vi "Init Loop Data.vi"(7 "VolatusAPI":refnum<class "VolatusAPI.lvclass">, 8 "error in (no error)":refnum<class "MultiErrors.lvclass">, 9 "Sequencer":refnum<class "MessageQ.lvclass">, 10 "Sequence Config":refnum<class "Sequence Config.lvclass">, 11 "Sequence in":refnum<class "Sequence.lvclass">) -> (0 "error out":refnum<class "MultiErrors.lvclass">, 2 "Loop Data":T1, 3 "Sequence out":refnum<class "Sequence.lvclass">, 5 "Period":i64)   [LabVIEW 2023, in "VolatusSeq.lvlib" / "Sequence.lvclass"]
uses:
  Sequence.lvclass
  VolatusErrorUtilities/MultiErrors/MultiErrors.lvclass
  VolatusSeqConfig/Sequence Config/Sequence Config.lvclass
  Loop Data.ctl
  Volatus/MessageQ/MessageQ.lvclass
  Sequence Time.ctl
  Volatus/VolatusAPI/VolatusAPI.lvclass
  VolatusErrorUtilities/MultiErrors/MultiErrors.lvclass/MultiErrors.ctl
  Sequence.lvclass/Sequence.ctl
  State/State.lvclass
  VolatusSeq.lvlib
  Variables/Variables.lvclass
  VolatusSeqConfig/Debug Flags.ctl
  VolatusSeqConfig/VolatusSeqConfig.lvlib
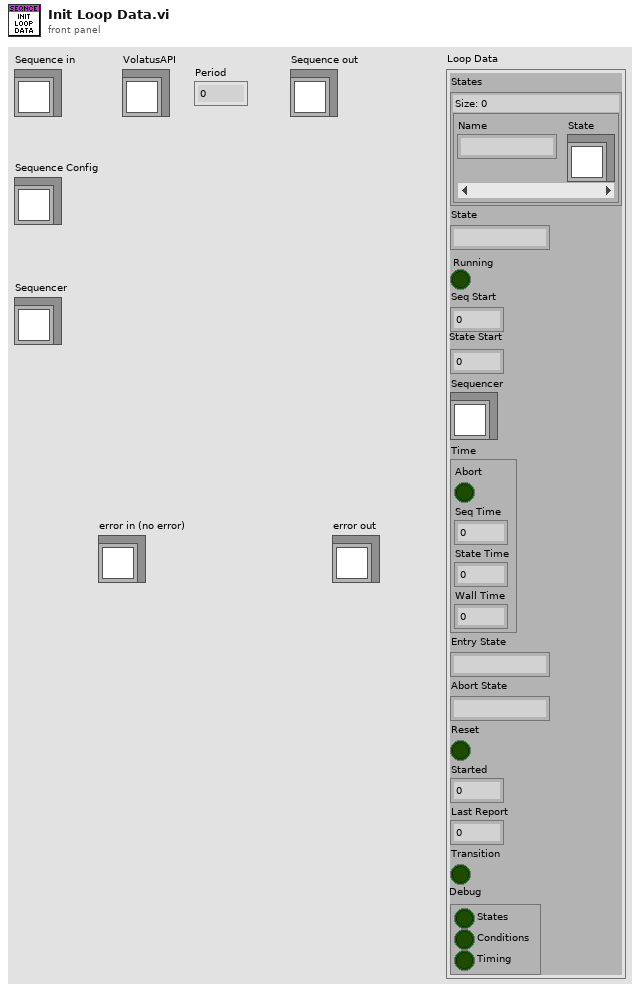
[diagram p1: front panel]
types:
  T1 = typedef "VolatusSeq.lvlib/Sequence.lvclass/Loop Data.ctl" = cluster{"States":map{string, refnum<class "State.lvclass">}, "State":string, "Running":bool, "Seq Start":dbl, "State Start":dbl, "Sequencer":refnum<class "MessageQ.lvclass">, "Time":T2, "Entry State":string, "Abort State":string, "Reset":bool, "Started":dbl, "Last Report":dbl, "Transition":bool, "Debug":T3}
  T2 = typedef "VolatusSeq.lvlib/Sequence Time.ctl" = cluster{"Abort":bool, "Seq Time":dbl, "State Time":dbl, "Wall Time":dbl}
  T3 = typedef "VolatusSeqConfig.lvlib/Debug Flags.ctl" = cluster{"States":bool, "Conditions":bool, "Timing":bool}
  T4 = typedef "VolatusSeq.lvlib/State Control.ctl" = cluster{"State":refnum<notifier>, "Time":refnum<notifier>, "Request State":refnum<notifier>, "Abort":refnum<notifier>, "Reset":refnum<notifier>, "Close":refnum<notifier>, "Vars SEQ":refnum<queue>}
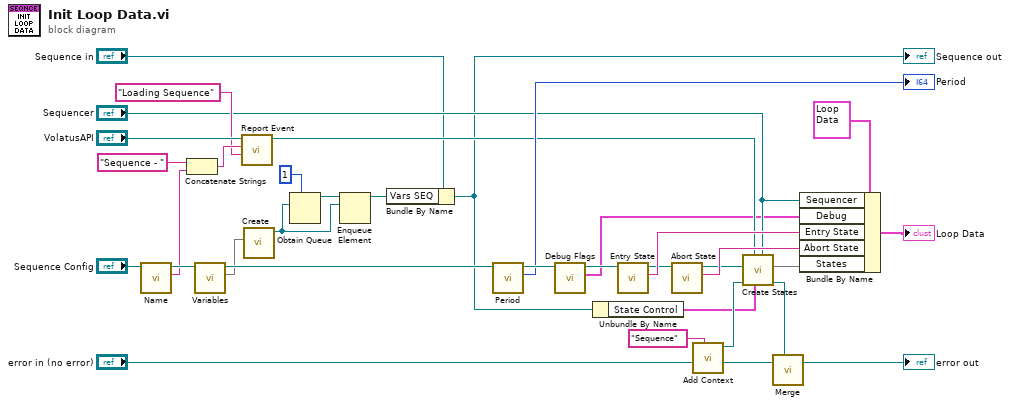
[diagram p0: block diagram]
diagram:
  n1 = call "Name.vi"("Sequence Config in"="Sequence Config") -> ("Name"=w14:string, "Sequence Config out"=w16:refnum<class "Sequence Config.lvclass">)  [unwired: 8 in, 1 out]
  n2 = Concatenate Strings("Sequence - ", w14) -> (w13:string)
  n3 = call "Variables.vi"("Sequence Config in"=w16) -> ("Variables"=w8:map{string, dbl}, "Sequence Config out"=w9:refnum<class "Sequence Config.lvclass">)  [unwired: 9 in]
  n4 = call "Report Event.vi"("Message"="Loading Sequence", "Context"=w13, "VolatusAPI in"="VolatusAPI") -> ("VolatusAPI out"=w18:refnum<class "VolatusAPI.lvclass">)  [unwired: 7 in, 1 out]
  n5 = call "Create.vi"("Variables"=w8) -> ("Variables out"=w5:refnum<class "Variables.lvclass">)  [unwired: 9 in, 1 out]
  n6 = Obtain Queue(max queue size (-1, unlimited)=1, element data type=w5) -> (queue out=w6:refnum<queue>)  [unwired: 3 in, 2 out]
  n7 = Enqueue Element(queue=w6, element=w5) -> (queue out=w2:refnum<queue>)  [unwired: 2 in, 2 out]
  n8 = Bundle By Name(cluster="Sequence in", "Vars SEQ"=w2) -> (w3:refnum<class "Sequence.lvclass">)
  "Sequence out" <- w3
  n9 = call "Period.vi"("Sequence Config in"=w9) -> ("Period"=→"Period":i64, "Sequence Config out"=w20:refnum<class "Sequence Config.lvclass">)  [unwired: 9 in]
  n10 = call "Debug Flags.vi"("Sequence Config in"=w20) -> ("Debug"=w1:T3, "Sequence Config out"=w10:refnum<class "Sequence Config.lvclass">)  [unwired: 9 in]
  n11 = Unbundle By Name(w3) -> ("State Control"=w30:T4)
  n12 = call "Entry State.vi"("Sequence Config in"=w10) -> ("Entry State"=w24:string, "Sequence Config out"=w23:refnum<class "Sequence Config.lvclass">)  [unwired: 9 in]
  n13 = call "Abort State.vi"("Sequence Config in"=w23) -> ("Abort State"=w22:string, "Sequence Config out"=w21:refnum<class "Sequence Config.lvclass">)  [unwired: 9 in]
  n14 = call "Add Context.vi"("Context"="Sequence", "MultiErrors in"="error in (no error)") -> ("Original Context"=w27:refnum<class "MultiErrors.lvclass">, "Added Context"=w35:refnum<class "MultiErrors.lvclass">)  [unwired: 8 in]
  n15 = call "Create States.vi"("Sequencer"="Sequencer", "State Control"=w30, "VolatusAPI"=w18, "error in (no error)"=w35, "Sequence Config"=w21) -> ("error out"=w25:refnum<class "MultiErrors.lvclass">, "States"=w31:map{string, refnum<class "State.lvclass">})  [unwired: 5 in]
  n16 = call "Merge.vi"("First Error In"=w27, "Second Error In"=w25) -> ("MultiErrors out"=→"error out":refnum<class "MultiErrors.lvclass">)  [unwired: 5 in]
  n17 = Bundle By Name(cluster=T1 {"States"={}, "State"="", "Running"=FALSE, "Seq Start"=0.0, "State Start"=0.0, "Sequencer"=refnum, "Time"={"Abort"=FALSE, "Seq Time"=0.0, "State Time"=0.0, "Wall Time"=0.0}, "Entry State"="", "Abort State"="", "Reset"=FALSE, "Started"=0.0, "Last Report"=0.0, "Transition"=FALSE, "Debug"={"States"=FALSE, "Conditions"=FALSE, "Timing"=FALSE}} ("Loop Data"), "Sequencer"="Sequencer", "Debug"=w1, "Entry State"=w24, "Abort State"=w22, "States"=w31) -> (→"Loop Data":T1)
